vi "Dialogue_String.vi"(7 "Empty String allowed?":bool=TRUE, 8 "error in":errorcluster, 11 "Title":string) -> (0 "error out":errorcluster, 2 "Cancelled?":bool=TRUE, 3 "Input":string)   [LabVIEW 2014, in "hse-ui.lvlib"]
doc: "Shows a dialog window for entering a string value.\n\n____\nHAMPEL SOFTWARE ENGINEERING v0.7.0 (2018-07-16 18:12)"
uses:
  hse-ui.lvlib
  FPControl/FPControl_Actions.ctl
panel:
  in  "Label":string caption="Enter Application Name"
  in  "Btn_Cancel":bool
  in  "Btn_OK":bool
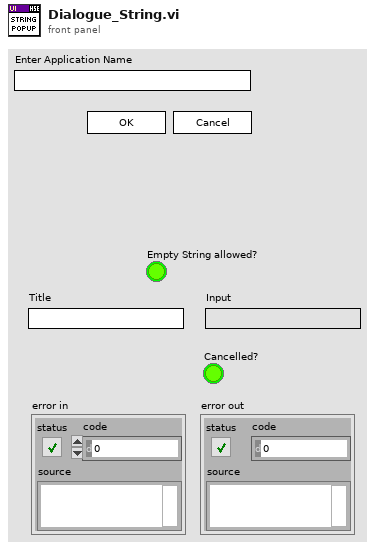
[diagram p1: front panel]
types:
  T1 = typedef "hse-ui.lvlib/FPControl_Actions.ctl" = enum16{"Open", "Hide", "Close", "Bring To Front", "Center", "Minimize", "Maximize"}
  T2 = enum8{"Enabled", "Disabled", "Disabled and Grayed Out"}
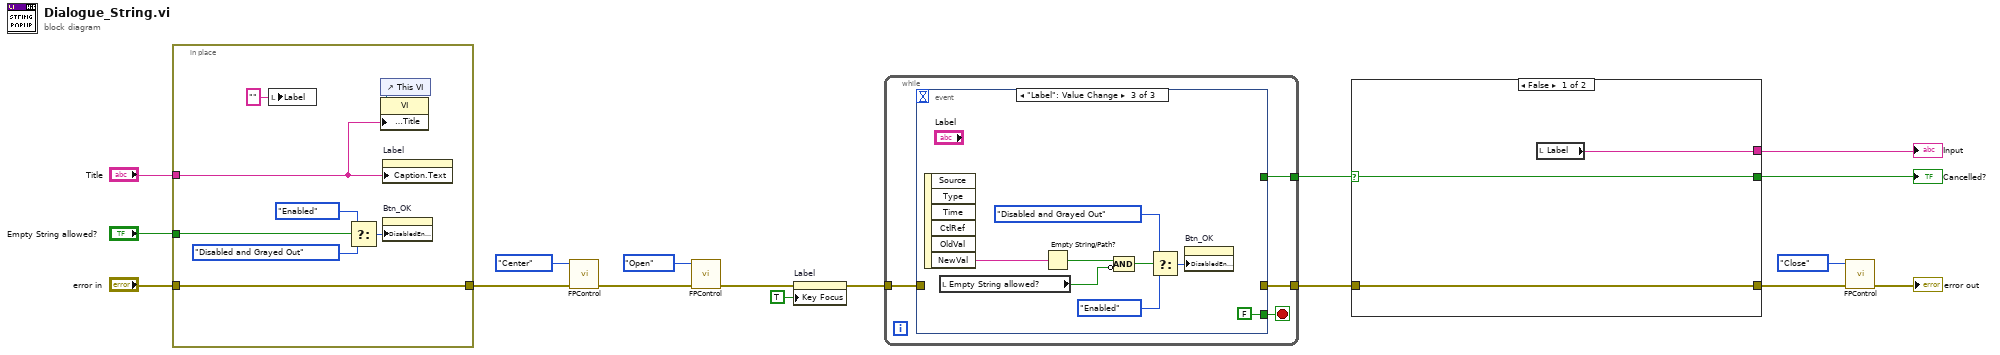
[diagram p0: block diagram]
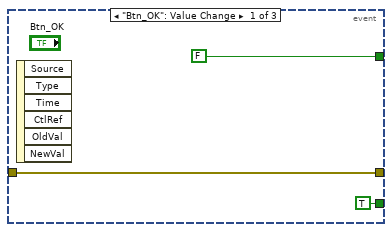
[diagram p2: hidden frame]
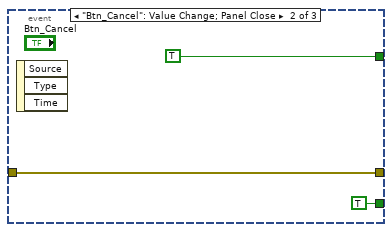
[diagram p3: hidden frame]
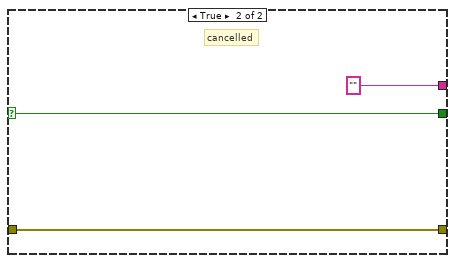
[diagram p4: hidden frame]
diagram:
  n1 = in-place {
    in-place-border: "error in" -> [w25]
    in-place-border: [w25] -> w7
    in-place-border: "Title" -> [w22]
    in-place-border: "Empty String allowed?" -> [w20]
    n2 = local write "Label"("" ("Label")) -> ()
    n3 = Select(t=T2."Enabled" ("Disabled"), s=w20, f=T2."Disabled and Grayed Out" ("Disabled")) -> (s? t:f=w19:T2)
    n4 = control-ref of="This VI"() -> (w23:refnum<vi>)
    n5 = property class="VI"(reference=w23, "Front Panel.Title"=w22) -> ()  [unwired: 1 in, 2 out]
    n6 = property on="Label" class="Str"("Caption.Text"=w22) -> ()  [unwired: 2 in, 2 out]
    n7 = property on="Btn_OK" class="Bool"("DisabledEnum"=w19) -> ()  [unwired: 2 in, 2 out]
  }
  n8 = call "FPControl.vi"("error in"=w7, "Function"=FPControl_Actions."Center") -> ("error out"=w15:errorcluster)  [unwired: 9 out]
  n9 = call "FPControl.vi"("error in"=w15, "Function"=FPControl_Actions."Open") -> ("error out"=w5:errorcluster)  [unwired: 9 out]
  n10 = property on="Label" class="Str"(error in=w5, "Key Focus"=TRUE) -> (error out=w4:errorcluster)  [unwired: 1 in, 1 out]
  n11 = while {
    tunnel: [w29] -> w12
    tunnel: [w28] -> w10
    tunnel: w4 -> [w27]
    stop <- w26 stop-if-true
    n12 = event shown="[2] \"Label\": Value Change" {
      selector: _ -> [_ _ _]
      dyn-events: _ -> [_ _ _]
      timeout: _ -> [_ _ _]
      tunnel: w27 -> [w32 w35 _]
      tunnel: [w32 w35 _] -> w29
      tunnel: [FALSE TRUE _] -> w28
      tunnel: [TRUE TRUE FALSE] -> w26
      event "Btn_OK": Value Change {
        n13 = event-data() -> ()  [unwired: 1 in, 6 out]
      }
      event "Btn_Cancel": Value Change; Panel Close {
        n14 = event-data() -> ()  [unwired: 1 in, 3 out]
      }
      event "Label": Value Change {
        n15 = event-data() -> ("NewVal"=w39:string)  [unwired: 1 in, 5 out]
        n16 = local read "Empty String allowed?"() -> (w36:bool)
        n17 = Empty String/Path?(string/path=w39) -> (empty?=w37:bool)
        n18 = Compound Arithmetic op=AND(w37, invert w36) -> (w38:bool)
        n19 = Select(t=T2."Disabled and Grayed Out" ("Disabled"), s=w38, f=T2."Enabled" ("Disabled")) -> (s? t:f=w42:T2)
        n20 = property on="Btn_OK" class="Bool"("DisabledEnum"=w42) -> ()  [unwired: 2 in, 2 out]
      }
    }
  }
  n21 = case shown="False" w10 {
    selector: w10 -> [w45 w47]
    tunnel: w12 -> [w46 w49]
    tunnel: [w46 w49] -> w11
    tunnel: [w44 ""] -> w9
    tunnel: [w45 w47] -> w2
    frame False {
      n22 = local read "Label"() -> (w44:string)
    }
    frame True {
      # "cancelled"
    }
  }
  "Input" <- w9
  "Cancelled?" <- w2
  n23 = call "FPControl.vi"("error in"=w11, "Function"=FPControl_Actions."Close") -> ("error out"=→"error out":errorcluster)  [unwired: 9 out]
